vi "TomsToolsDocumentationTool_Provider_OnCommand.vi"(10 "Command ID":string, 11 "objects":T1[](array[typedef])) -> ()   [LabVIEW 2015]
uses:
  <resource>/Framework/Providers/API/ItemRef.ctl
  Model Messages/Add VI from File Msg/Add VI from File Msg.lvclass/Add VI from File Msg.ctl
  <vilib>/ActorFramework/Message Enqueuer/Message Enqueuer.lvclass/Message Enqueuer.ctl
  <vilib>/ActorFramework/Message Enqueuer/Enqueue.vi
  <vilib>/ActorFramework/Message Priority Queue/Priority Enqueue.vi
  Model Messages/Add VI from File Msg/Add VI from File Msg.lvclass
panel:
  out "error out":errorcluster
  in  "error in":errorcluster
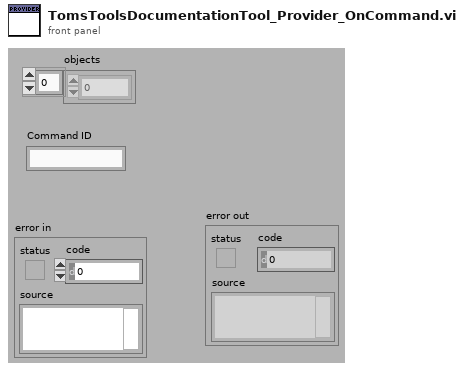
[diagram p1: front panel]
types:
  T1 = typedef "ItemRef.ctl" = u64
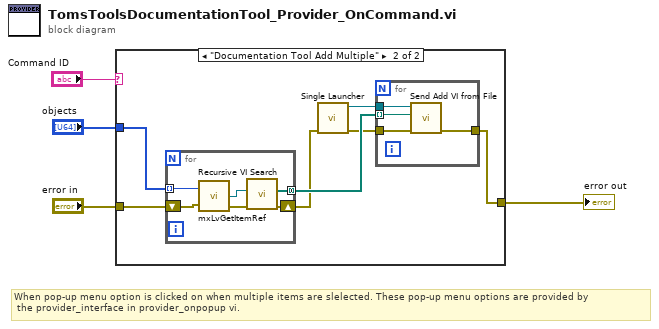
[diagram p0: block diagram]
diagram:
  # "When pop-up menu option is clicked on when multiple items are slelected. These pop-up menu options are provided by\n the provider_interface in provider_onpopup vi."
  n1 = case shown="\"Documentation Tool Add Multiple\"" "Command ID" {
    tunnel: "objects" -> [_ w12]
    tunnel: "error in" -> [w5 w11]
    tunnel: [w5 w6] -> w1
    frame Default {
    }
    frame "Documentation Tool Add Multiple" {
      n2 = for {
        tunnel: w12 -> [w22] mode=indexing
        shift-right: [w19] -> w7
        shift-left: w11 -> [w21]
        tunnel: [w18] -> w9 mode=concatenating
        n3 = call <resource>:"mxLvGetItemRef.vi"("Item"=w22, "error in"=w21) -> ("Item Refnum"=w17:refnum<vi>, "error out"=w20:errorcluster)  [unwired: 1 out]
        n4 = call "Recursive VI Search.vi"("error in (no error)"=w20, "Project Item"=w17) -> ("error out"=w19:errorcluster, "VI Paths"=w18:path[])  [unwired: 8 in]
      }
      n5 = call "Single Launcher.vi"("error in (no errors)"=w7) -> ("error out"=w8:errorcluster, "Documentation Tool Model"=w10:refnum<class "Message Enqueuer.lvclass">)  [unwired: 9 in]
      n6 = for {
        tunnel: w10 -> [w16]
        tunnel: w9 -> [w15] mode=indexing
        tunnel: w8 -> [w14]
        tunnel: [w13] -> w6
        n7 = call "Send Add VI from File.vi"("error in (no error)"=w14, "VI Path"=w15, "Message Enqueuer"=w16) -> ("error out"=w13:errorcluster)  [unwired: 7 in, 1 out]
      }
    }
  }
  "error out" <- w1
